vi "MGI Bezier Vector (DBL).vi"(2 "u":dbl format="%.2f", 3 "First k":i32, 4 "Bezier Control Points[k][dims]":dbl[][](array[numeric]) format="%.2f") -> (0 "Bezier Weights[]":dbl[](array[numeric]) format="%.2f", 1 "N-dimensional Vector[]":dbl[](array[numeric]) format="%.2f")   [LabVIEW 2016]
doc: "Compute an N-Dimensional Bezier vector given sets of 4 control points in each of N dimensions and the desired 0-1 value.\n\nAuthored by David A. Moore\nsupport@mooregoodideas.com\nwww.mooregoodideas.com\n\nCopyright (c) 2010, Moore Good Ideas, Inc.\n\nAll rights reserved.\n\nRedistribution and use in source and binary forms, with or without modification, are permitted provided that the following conditions are met:\n\n * Redistributions of source code must retain the above copyright notice, this list of conditions and the following disclaimer.\n * Redistributions in binary form must reproduce the above copyright notice, this list of conditions and the following disclaimer in the documentation and/or other materials provided with the distribution.\n * Neither the name of Moore Good Ideas, Inc. nor the names of its contributors may be used to endorse or promote products derived from this software without specific prior written permission.\n\nTHIS SOFTWARE IS PROVIDED BY THE COPYRIGHT HOLDERS AND CONTRIBUTORS \"AS IS\" AND ANY EXPRESS OR IMPLIED WARRANTIES, INCLUDING, BUT NOT LIMITED TO, THE IMPLIED WARRANTIES OF MERCHANTABILITY AND FITNESS FOR A PARTICULAR PURPOSE ARE DISCLAIMED. IN NO EVENT SHALL THE COPYRIGHT OWNER OR CONTRIBUTORS BE LIABLE FOR ANY DIRECT, INDIRECT, INCIDENTAL, SPECIAL, EXEMPLARY, OR CONSEQUENTIAL DAMAGES (INCLUDING, BUT NOT LIMITED TO, PROCUREMENT OF SUBSTITUTE GOODS OR SERVICES; LOSS OF USE, DATA, OR PROFITS; OR BUSINESS INTERRUPTION) HOWEVER CAUSED AND ON ANY THEORY OF LIABILITY, WHETHER IN CONTRACT, STRICT LIABILITY, OR TORT (INCLUDING NEGLIGENCE OR OTHERWISE) ARISING IN ANY WAY OUT OF THE USE OF THIS SOFTWARE, EVEN IF ADVISED OF THE POSSIBILITY OF SUCH DAMAGE."
uses:
  <userlib>/_MGI/Bezier/MGI Bezier Weights/MGI Bezier Weights (DBL).vi
panel:
  # "k"
  # "dims"
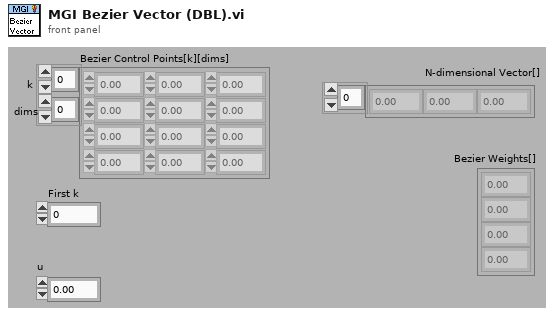
[diagram p1: front panel]
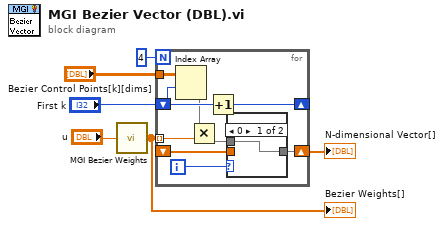
[diagram p0: block diagram]
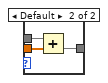
[diagram p2: hidden frame]
diagram:
  n1 = call-poly <userlib>:"MGI Bezier Weights.vi"("u"="u") -> ("Bezier Weights"=w4:dbl[])
  "Bezier Weights[]" <- w4
  n2 = for {
    N: 4 -> [_]
    tunnel: w4 -> [w11] mode=indexing
    tunnel: "Bezier Control Points[k][dims]" -> [w9]
    shift-right: [w14] -> w3
    shift-left: _ -> [w13]
    shift-right: [w8] -> _
    shift-left: "First k" -> [w10]
    i -> [w12]
    n3 = Index Array(array=w9, index (row)=w10) -> (element=w7:dbl[])  [unwired: 1 in]
    n4 = Multiply(x=w7, y=w11) -> (x*y=w15:dbl[])
    n5 = Increment(x=w10) -> (x+1=w8:i32)
    n6 = case shown="0" w12 {
      tunnel: w15 -> [w16 w19]
      tunnel: [w16 w18] -> w14
      tunnel: w13 -> [_ w17]
      frame 0 {
      }
      frame Default {
        n7 = Add(x=w19, y=w17) -> (x+y=w18:dbl[])
      }
    }
  }
  "N-dimensional Vector[]" <- w3
